vi "SQL_configuration_select_table.vi"() -> (2 "error out":errorcluster, 3 "表格控件":string[][](table))   [LabVIEW 2014]
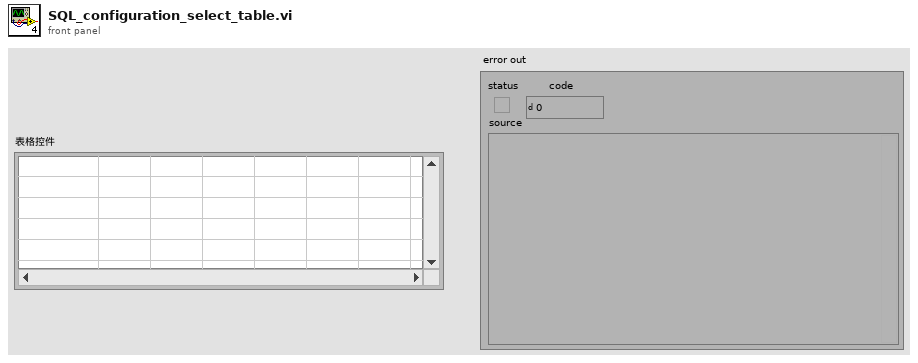
[diagram p1: front panel]
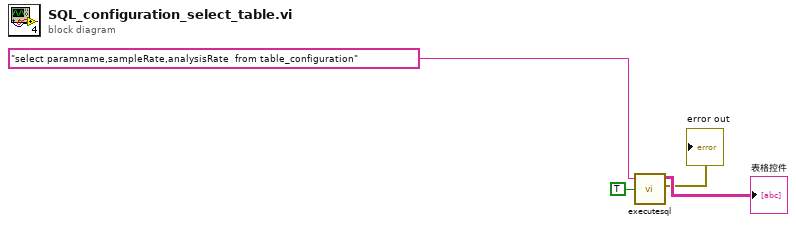
[diagram p0: block diagram]
diagram:
  n1 = call "executesql.vi"("Return Data (T)"=TRUE, "Command Text"="select paramname,sampleRate,analysisRate  from table_configuration") -> ("error out"=→"error out":errorcluster, "Data"=→"表格控件":string[][])  [unwired: 5 in]
